vi "FormUserManagement.vi"() -> ()   [LabVIEW 2012]
uses:
  <vilib>/addons/database/_DB Variant To Data/Database Variant To Data.xnode
panel:
  in  "更新":bool
  in  "设备管理员":bool
  in  "有效用户":bool
  in  "编号":string
  in  "用户":string(combo)
  out "表格控件":string[][](table) caption="已注册用户"
  in  "删除":bool
  in  "注册":bool
  in  "密码":string
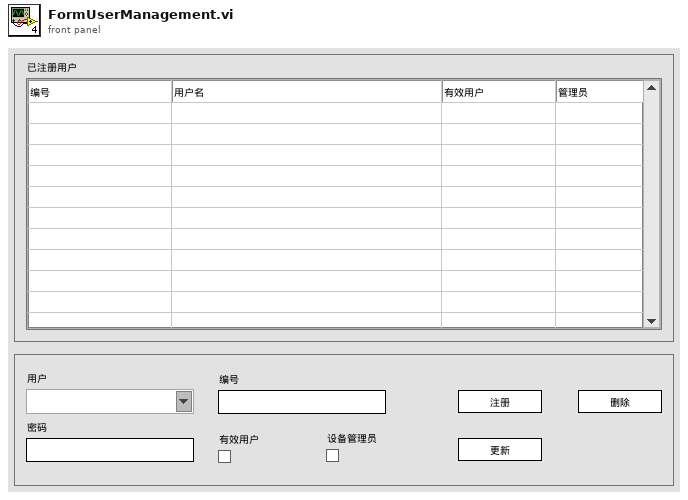
[diagram p1: front panel]
types:
  T1 = enum8{"Enabled", "Disabled", "Disabled and Grayed Out"}
  T2 = cluster{"userCode":string, "userName":string, "userStatus":string, "connectionMode":string, "takesTime":string, "countDone":string, "countOK":string, "countNG":string, "rigStatus":string, "productsName":string, "partCode1":string, "partCode2":string, "partCode3":string}
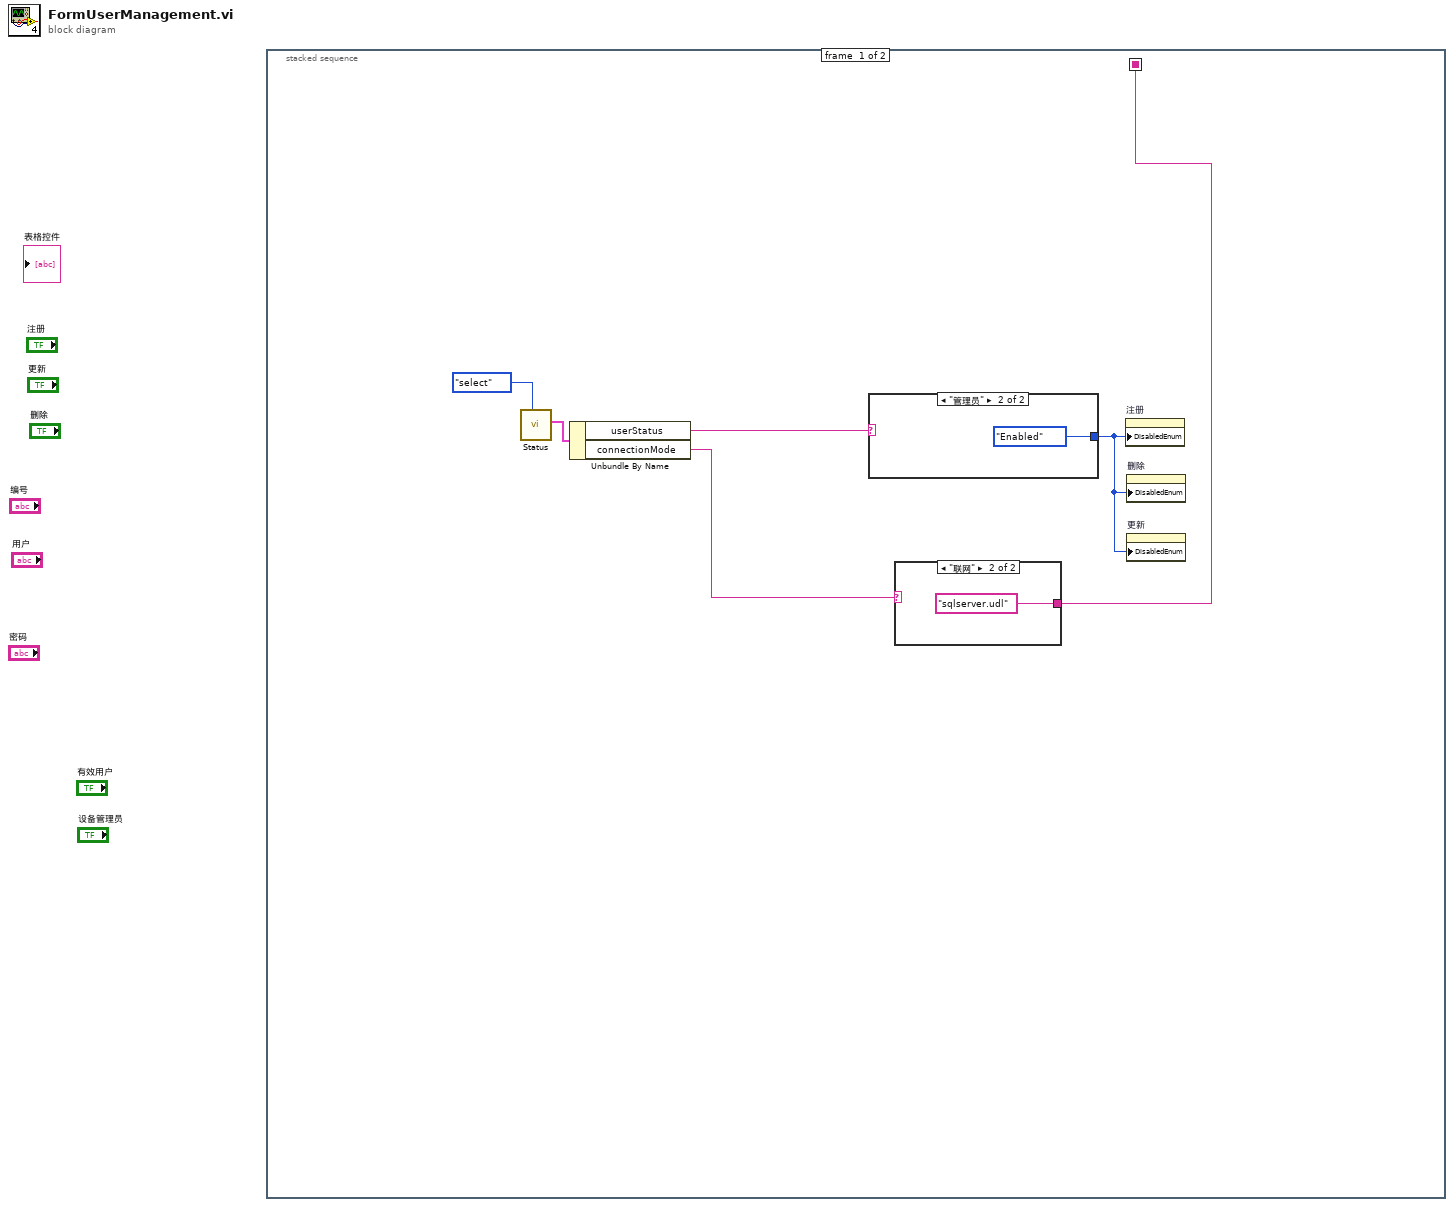
[diagram p0: block diagram]
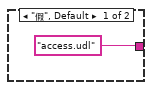
[diagram p2: hidden frame]
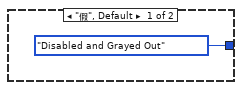
[diagram p3: hidden frame]
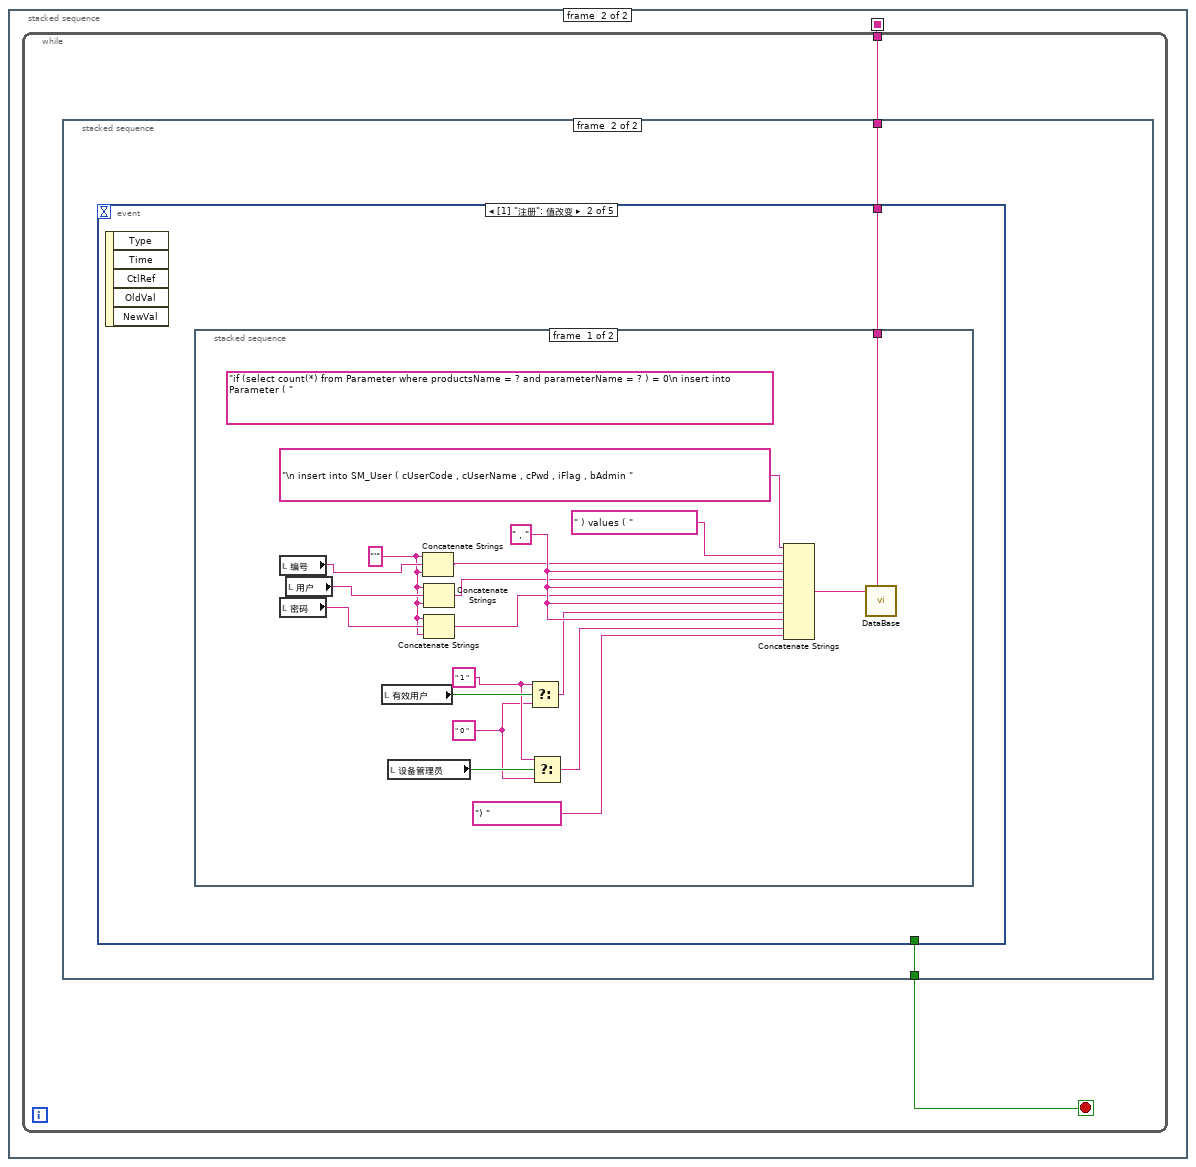
[diagram p4: hidden frame]
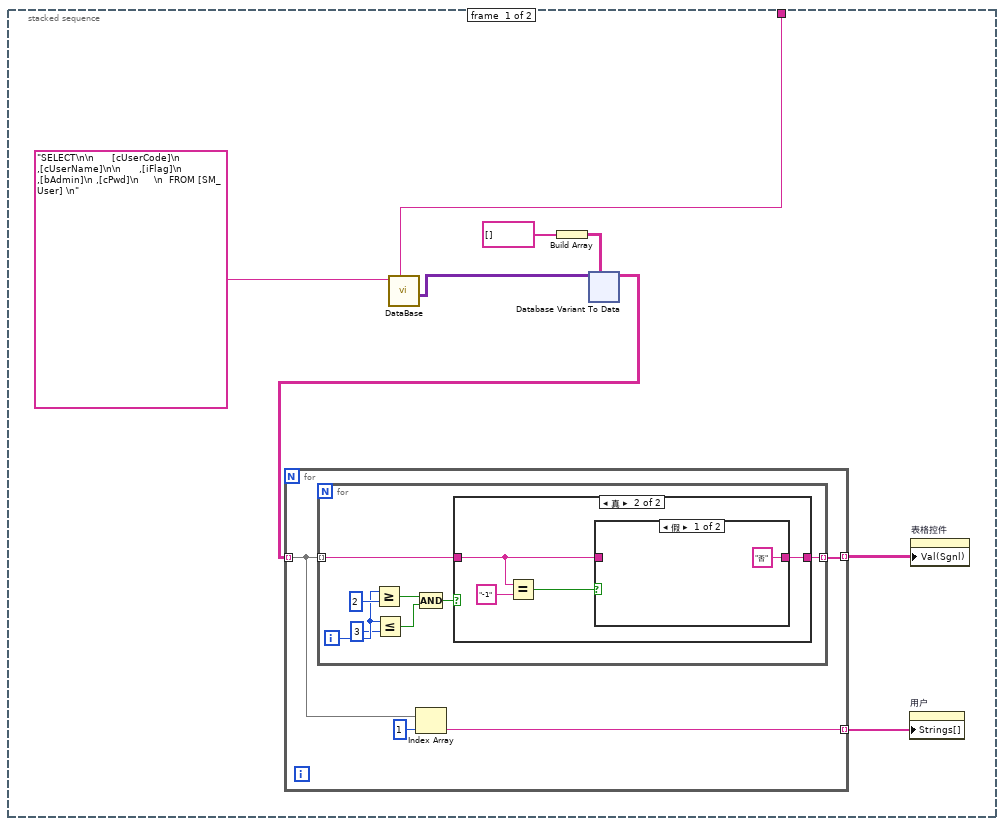
[diagram p5: hidden frame]
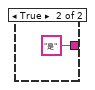
[diagram p7: hidden frame]
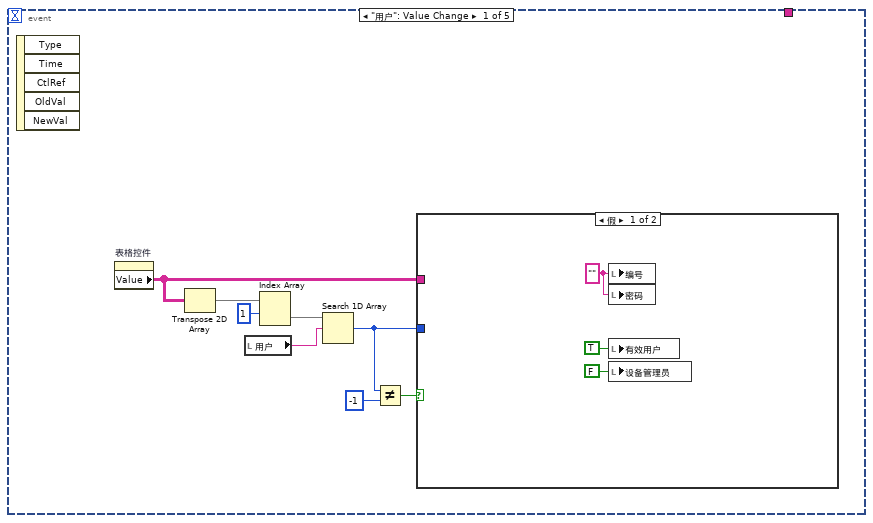
[diagram p8: hidden frame]
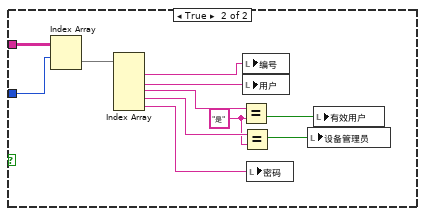
[diagram p9: hidden frame]
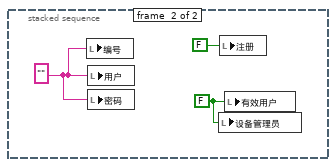
[diagram p10: hidden frame]
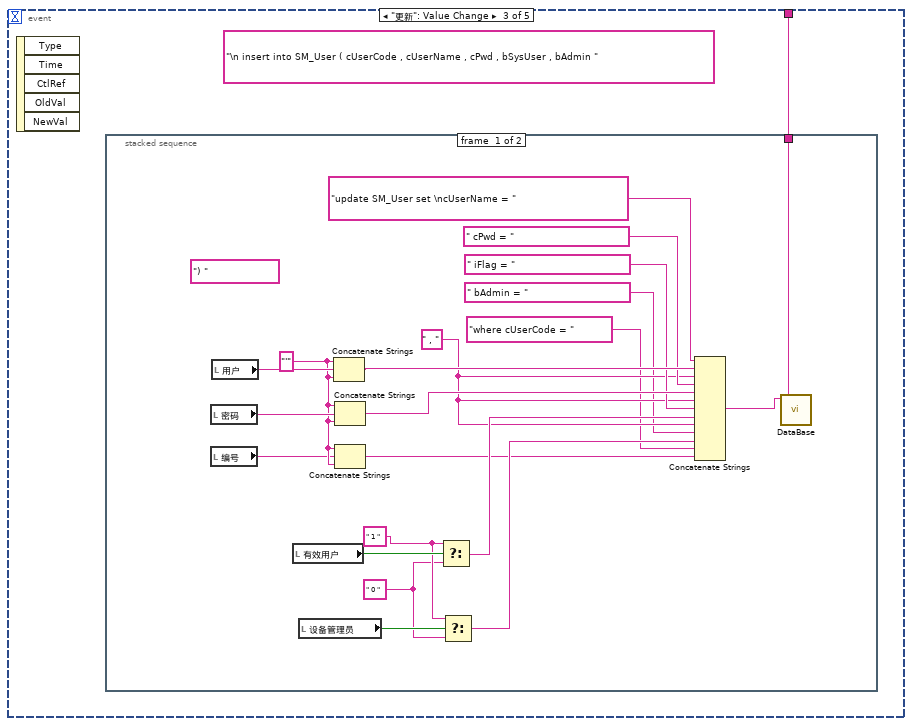
[diagram p11: hidden frame]
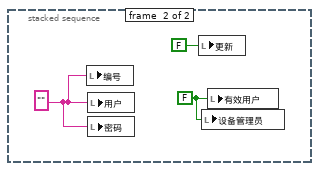
[diagram p12: hidden frame]
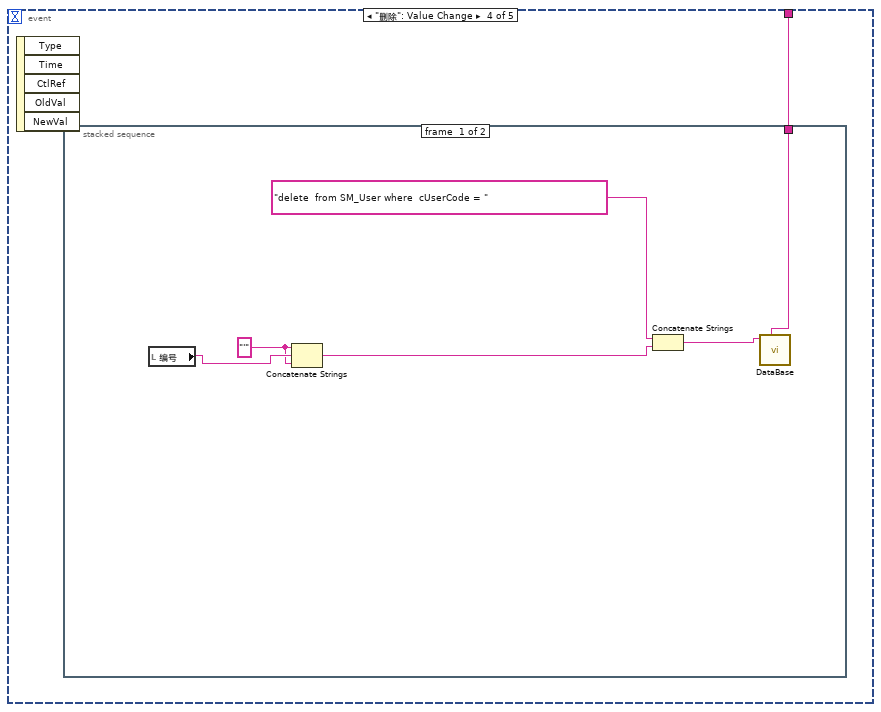
[diagram p13: hidden frame]
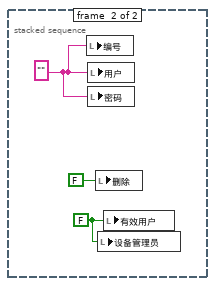
[diagram p14: hidden frame]
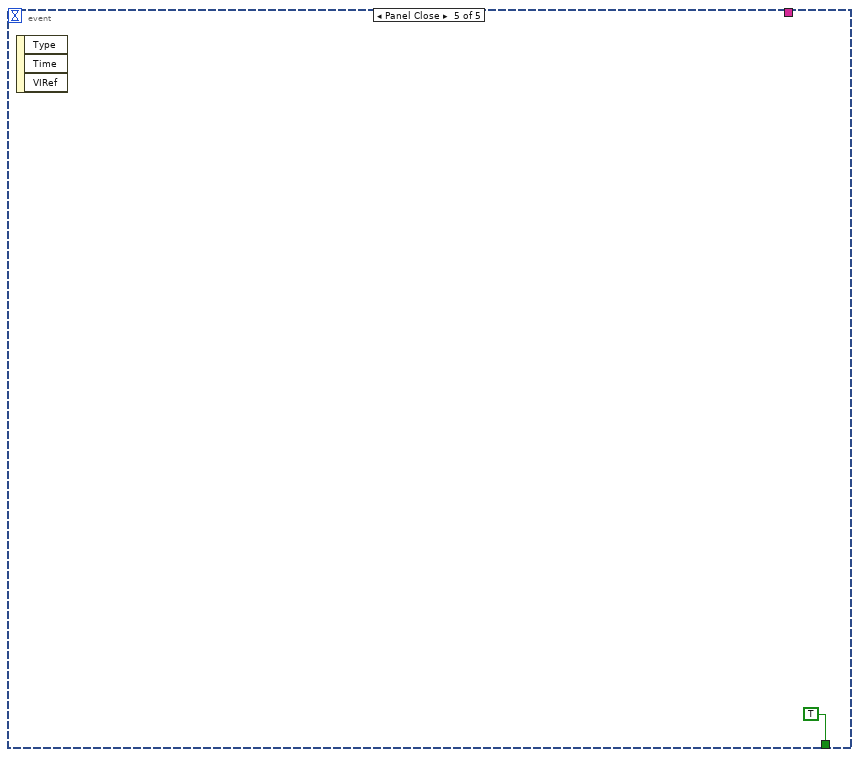
[diagram p15: hidden frame]
diagram:
  n1 = stacked-sequence {
    seq-local: [w1 _] -> [_ w11]
    frame #0 {
      n2 = call "Status.vi"("模式"=enum16{"select", "insert", "update", "delete"}."select") -> ("元素"=w5:T2)  [unwired: 10 in]
      n3 = Unbundle By Name(w5) -> ("userStatus"=w3:string, "connectionMode"=w2:string)
      n4 = case shown="\"管理员\"" w3 {
        tunnel: [T1."Disabled and Grayed Out" ("禁用") T1."Enabled" ("禁用")] -> w6
        frame "假", Default {
        }
        frame "管理员" {
        }
      }
      n5 = case shown="\"联网\"" w2 {
        tunnel: ["access.udl" ("udl名称") "sqlserver.udl" ("udl名称")] -> w1
        frame "假", Default {
        }
        frame "联网" {
        }
      }
      n6 = property on="注册" class="Bool (严格)"("DisabledEnum"=w6) -> ()  [unwired: 2 in, 2 out]
      n7 = property on="删除" class="Bool (严格)"("DisabledEnum"=w6) -> ()  [unwired: 2 in, 2 out]
      n8 = property on="更新" class="Bool (严格)"("DisabledEnum"=w6) -> ()  [unwired: 2 in, 2 out]
    }
    frame #1 {
      n9 = while {
        tunnel: w11 -> [w12]
        stop <- w13 stop-if-true
        n10 = stacked-sequence {
          tunnel: [_ w86] -> w13
          tunnel: w12 -> [w14 w85]
          frame #0 {
            n11 = call "DataBase.vi"("udl名称"=w14, "SQL query"="SELECT\n\n      [cUserCode]\n      ,[cUserName]\n\n      ,[iFlag]\n      ,[bAdmin]\n ,[cPwd]\n     \n  FROM [SM_User] \n") -> ("recordset data"=w18:variant[][])  [unwired: 9 in]
            n12 = Build Array(string[] [] ("添加的数组")) -> (w19:string[][])
            n13 = xnode "Database Variant To Data"("database variant"=w18, "type"=w19) -> ("data"=w17:string[][])  [unwired: 1 in, 1 out]
            n14 = for {
              tunnel: w17 -> [w24] mode=indexing
              tunnel: [w25] -> w16 mode=indexing
              tunnel: [w22] -> w15 mode=indexing
              n15 = for {
                tunnel: w24 -> [w32] mode=indexing
                tunnel: [w31] -> w25 mode=indexing
                i -> [w27]
                n16 = Greater Or Equal?(x=w27, y=2) -> (x >= y?=w29:bool)
                n17 = Less Or Equal?(x=w27, y=3) -> (x <= y?=w28:bool)
                n18 = Compound Arithmetic op=AND(w29, w28) -> (w30:bool)
                n19 = case shown="真" w30 {
                  tunnel: w32 -> [w34 w35]
                  tunnel: [w34 w36] -> w31
                  frame False {
                  }
                  frame True {
                    n20 = Equal?(x=w35, y="-1") -> (x = y?=w37:bool)
                    n21 = case shown="假" w37 {
                      tunnel: ["否" ("字符串") "是" ("字符串")] -> w36
                      tunnel: w35 -> [_ _]
                      frame False {
                      }
                      frame True {
                      }
                    }
                  }
                }
              }
              n22 = Index Array(array=w24, index=1 ("索引")) -> (element=w22:string)
            }
            n23 = property on="用户" class="CmbBox"("Strings[]"=w15) -> ()  [unwired: 2 in, 2 out]
            n24 = property on="表格控件" class="Tbl (严格)"("Val(Sgnl)"=w16) -> ()  [unwired: 2 in, 2 out]
          }
          frame #1 {
            n25 = event shown="[1] \"注册\": 值改变" {
              selector: _ -> [_ _ _ _ _]
              dyn-events: _ -> [_ _ _ _ _]
              timeout: _ -> [_ _ _ _ _]
              tunnel: [_ _ _ _ TRUE] -> w86
              tunnel: w85 -> [_ w109 w132 w157 _]
              event "用户": Value Change {
                n26 = event-data() -> ()  [unwired: 1 in, 5 out]
                n27 = property on="表格控件" class="Tbl (严格)"() -> ("Value"=w90:string[][])  [unwired: 2 in, 2 out]
                n28 = Transpose 2D Array(2D array=w90) -> (transposed array=w94:string[][])
                n29 = local read "用户"() -> (w91:string)
                n30 = Index Array(array=w94, index (row)=1 ("索引 (行)")) -> (element=w92:string[])  [unwired: 1 in]
                n31 = Search 1D Array(1D array=w92, element=w91) -> (index of element=w87:i32)  [unwired: 1 in]
                n32 = Not Equal?(x=w87, y=-1) -> (x != y?=w89:bool)
                n33 = case shown="假" w89 {
                  tunnel: w90 -> [_ w108]
                  tunnel: w87 -> [_ w98]
                  frame False {
                    w95 = "" ("编号")
                    n34 = local write "编号"(w95) -> ()
                    n35 = local write "密码"(w95) -> ()
                    n36 = local write "有效用户"(TRUE ("有效用户")) -> ()
                    n37 = local write "设备管理员"(FALSE ("设备管理员")) -> ()
                  }
                  frame True {
                    w102 = "是" ("y")
                    n38 = Index Array(array=w108, index (row)=w98) -> (element=w107:string[])  [unwired: 1 in]
                    n39 = Index Array(array=w107) -> (element #1=w106:string, element #2=w105:string, element #3=w104:string, element #4=w103:string, element #5=w99:string)  [unwired: 5 in]
                    n40 = Equal?(x=w104, y=w102) -> (x = y?=w101:bool)
                    n41 = Equal?(x=w103, y=w102) -> (x = y?=w100:bool)
                    n42 = local write "编号"(w106) -> ()
                    n43 = local write "用户"(w105) -> ()
                    n44 = local write "密码"(w99) -> ()
                    n45 = local write "设备管理员"(w100) -> ()
                    n46 = local write "有效用户"(w101) -> ()
                  }
                }
              }
              event "注册": Value Change {
                n47 = event-data() -> ()  [unwired: 1 in, 5 out]
                n48 = stacked-sequence {
                  tunnel: w109 -> [w110 _]
                  frame #0 {
                    w112 = "'"
                    w123 = " 0 "
                    w124 = " 1 "
                    w122 = " , "
                    (unwired) "if (select count(*) from Parameter where productsName = ? and parameterName = ? ) = 0\n insert into Parameter ( " ("SQL query")
                    n49 = local read "编号"() -> (w118:string)
                    n50 = local read "密码"() -> (w114:string)
                    n51 = local read "用户"() -> (w116:string)
                    n52 = local read "有效用户"() -> (w126:bool)
                    n53 = local read "设备管理员"() -> (w125:bool)
                    n54 = Concatenate Strings(w112, w118, w112) -> (w117:string)
                    n55 = Concatenate Strings(w112, w116, w112) -> (w115:string)
                    n56 = Concatenate Strings(w112, w114, w112) -> (w113:string)
                    n57 = Select(t=w124, s=w126, f=w123) -> (s? t:f=w121:string)
                    n58 = Select(t=w124, s=w125, f=w123) -> (s? t:f=w120:string)
                    n59 = Concatenate Strings("\n insert into SM_User ( cUserCode , cUserName , cPwd , iFlag , bAdmin " ("SQL query"), " ) values ( " ("SQL query"), w117, w122, w115, w122, w113, w122, w121, w122, w120, ") " ("SQL query")) -> (w111:string)
                    n60 = call "DataBase.vi"("udl名称"=w110, "SQL query"=w111) -> ()  [unwired: 9 in, 1 out]
                  }
                  frame #1 {
                    w129 = FALSE ("系统管理员")
                    w131 = ""
                    n61 = local write "编号"(w131) -> ()
                    n62 = local write "用户"(w131) -> ()
                    n63 = local write "密码"(w131) -> ()
                    n64 = local write "设备管理员"(w129) -> ()
                    n65 = local write "注册"(FALSE ("注册")) -> ()
                    n66 = local write "有效用户"(w129) -> ()
                  }
                }
              }
              event "更新": Value Change {
                (unwired) "\n insert into SM_User ( cUserCode , cUserName , cPwd , bSysUser , bAdmin " ("SQL query")
                n67 = event-data() -> ()  [unwired: 1 in, 5 out]
                n68 = stacked-sequence {
                  tunnel: w132 -> [w133 _]
                  frame #0 {
                    w137 = "'"
                    w150 = " 0 "
                    w151 = " 1 "
                    w141 = " , "
                    (unwired) ") " ("SQL query")
                    n69 = local read "密码"() -> (w148:string)
                    n70 = local read "编号"() -> (w136:string)
                    n71 = local read "用户"() -> (w146:string)
                    n72 = local read "有效用户"() -> (w153:bool)
                    n73 = local read "设备管理员"() -> (w152:bool)
                    n74 = Concatenate Strings(w137, w146, w137) -> (w149:string)
                    n75 = Concatenate Strings(w137, w148, w137) -> (w144:string)
                    n76 = Concatenate Strings(w137, w136, w137) -> (w135:string)
                    n77 = Select(t=w151, s=w153, f=w150) -> (s? t:f=w142:string)
                    n78 = Select(t=w151, s=w152, f=w150) -> (s? t:f=w139:string)
                    n79 = Concatenate Strings("update SM_User set \ncUserName = " ("SQL query"), w149, w141, " cPwd = " ("SQL query"), w144, w141, " iFlag = " ("SQL query"), w142, w141, " bAdmin = " ("SQL query"), w139, "where cUserCode = " ("SQL query"), w135) -> (w134:string)
                    n80 = call "DataBase.vi"("udl名称"=w133, "SQL query"=w134) -> ()  [unwired: 9 in, 1 out]
                  }
                  frame #1 {
                    w154 = FALSE ("系统管理员")
                    w156 = ""
                    n81 = local write "编号"(w156) -> ()
                    n82 = local write "用户"(w156) -> ()
                    n83 = local write "密码"(w156) -> ()
                    n84 = local write "更新"(FALSE ("注册")) -> ()
                    n85 = local write "设备管理员"(w154) -> ()
                    n86 = local write "有效用户"(w154) -> ()
                  }
                }
              }
              event "删除": Value Change {
                n87 = event-data() -> ()  [unwired: 1 in, 5 out]
                n88 = stacked-sequence {
                  tunnel: w157 -> [w159 _]
                  frame #0 {
                    w162 = "'"
                    n89 = local read "编号"() -> (w163:string)
                    n90 = Concatenate Strings(w162, w163, w162) -> (w158:string)
                    n91 = Concatenate Strings("delete  from SM_User where  cUserCode = " ("SQL query"), w158) -> (w160:string)
                    n92 = call "DataBase.vi"("udl名称"=w159, "SQL query"=w160) -> ()  [unwired: 9 in, 1 out]
                  }
                  frame #1 {
                    w164 = FALSE ("系统管理员")
                    w166 = ""
                    n93 = local write "编号"(w166) -> ()
                    n94 = local write "用户"(w166) -> ()
                    n95 = local write "密码"(w166) -> ()
                    n96 = local write "删除"(FALSE ("删除")) -> ()
                    n97 = local write "设备管理员"(w164) -> ()
                    n98 = local write "有效用户"(w164) -> ()
                  }
                }
              }
              event Panel Close {
                n99 = event-data() -> ()  [unwired: 1 in, 3 out]
              }
            }
          }
        }
      }
    }
  }
